vi "PCO_GetHWIOSignalTiming.vi"(0 "ph":u64, 5 "error in (no error)":errorcluster {"code" format="%x"}) -> (14 "ph out":u64, 15 "ErrorMessage":i32 format="%x", 16 "wSignalNum":u16, 17 "wSelect":u16, 18 "dwSignalTiming":u32, 19 "error out":errorcluster {"code" format="%x"})   [LabVIEW 2019, in "SDK.lvlib" / "TimingControl.lvlib"]
doc: "<b>Description:</b>\nGets the signal timing and selected signal functionality of the requested signal number\nThis function call is optional. Please check camera description.\n\n<b>Supported camera type:</b>\npco.edge, pco.dimax\n\n<b>Descriptor dependency:</b>\ndwGeneralCapsDESC1: HW_IO_SIGNAL_DESCRIPTOR"
uses:
  TimingControl.lvlib
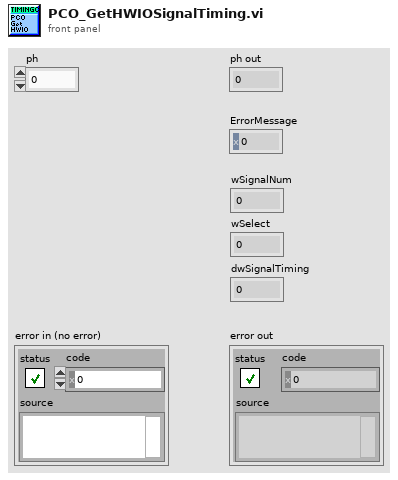
[diagram p1: front panel]
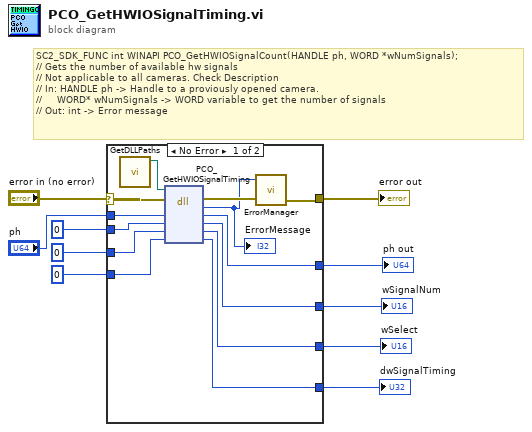
[diagram p0: block diagram]
diagram:
  # "SC2_SDK_FUNC int WINAPI PCO_GetHWIOSignalCount(HANDLE ph, WORD *wNumSignals);\n// Gets the number of available hw signals\n// Not applicable to all cameras. Check Description\n// In: HANDLE ph -> Handle to a proviously opened camera.\n//     WORD* wNumSignals -> WORD variable to get the number of signals\n// Out: int -> Error message"
  n1 = case shown="No Error" "error in (no error)" {
    selector: "error in (no error)" -> [w16 w28]
    tunnel: "ph" -> [w23 w27]
    tunnel: [w22 w27] -> w9
    tunnel: u16 0 ("wNumSignals") -> [w21 w26]
    tunnel: [w20 w26] -> w7
    tunnel: [w18 w28] -> w6
    tunnel: u16 0 ("wNumSignals") -> [w14 w25]
    tunnel: u32 0 ("wNumSignals") -> [w13 w24]
    tunnel: [w12 w25] -> w2
    tunnel: [w11 w24] -> w1
    frame No Error {
      n2 = call "GetDLLPaths.vi"() -> ("SC2_Cam_Path"=w15:path)  [unwired: 8 in, 3 out]
      n3 = dll-call lib="?" fn="PCO_GetHWIOSignalTiming"(path in=w15, error in=w16, "ph"=w23, "pwSignalNum"=w21, "pwSelect"=w14, "pdwSignalTiming"=w13) -> (error out=w19:errorcluster, "return type"=w17:i32, "ph"=w22:u64, "pwSignalNum"=w20:u16, "pwSelect"=w12:u16, "pdwSignalTiming"=w11:u32)  [unwired: 1 in, 1 out]
      "ErrorMessage" <- w17
      n4 = call "ErrorManager.vi"("error in (no error)"=w19, "error code"=w17) -> ("error out"=w18:errorcluster)  [unwired: 2 in, 1 out]
    }
    frame Error {
    }
  }
  "ph out" <- w9
  "wSignalNum" <- w7
  "error out" <- w6
  "wSelect" <- w2
  "dwSignalTiming" <- w1
